vi "Dash_Globals.vi"() -> ()   [LabVIEW 2023]
panel:
  out "Robot Mode":T1(ring)
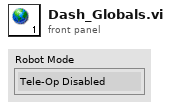
[diagram p1: front panel]
types:
  T1 = enum8{"Tele-Op Disabled", "Tele-Op Enabled", "Auto Disabled", "Auto Enabled", "Test Disabled", "Test Enabled", "Disconnected", "No Code", "E-Stop"}
diagram:
